vi "WRITE_P.vi"(8 "error in (no error)":errorcluster, 10 "productos 2":T1(array[cluster])) -> (0 "error out":errorcluster)   [LabVIEW 2020, in "Productos.lvlib"]
uses:
  Productos.lvlib
  <vilib>/Utility/xml.llb/Write to XML File(string).vi
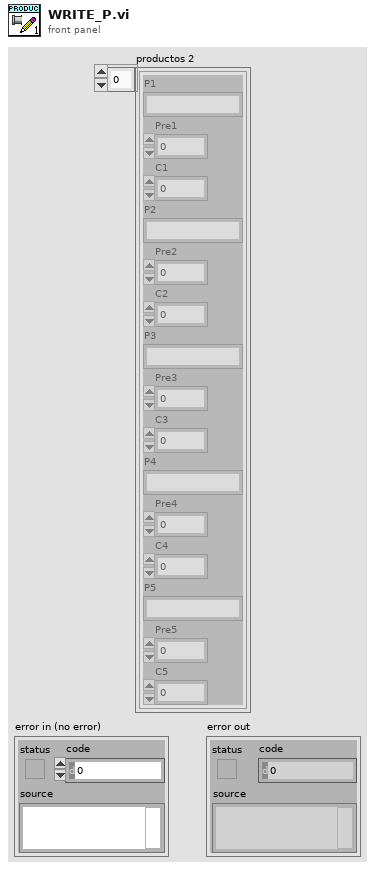
[diagram p1: front panel]
types:
  T1 = cluster{"P1":string, "Pre1":dbl, "C1":dbl, "P2":string, "Pre2":dbl, "C2":dbl, "P3":string, "Pre3":dbl, "C3":dbl, "P4":string, "Pre4":dbl, "C4":dbl, "P5":string, "Pre5":dbl, "C5":dbl}[]
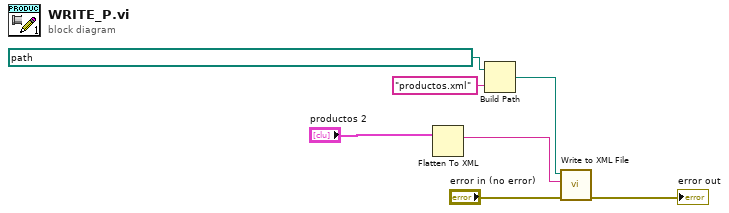
[diagram p0: block diagram]
diagram:
  n1 = Flatten To XML(6:"productos 2") -> (2:w5:string)
  n2 = Build Path(base path=path "C:/Users/Ymata/Desktop/séptimo/labview 7mo/Proyecto máuina/Proyecto-maquina", name or relative path="productos.xml") -> (appended path=w2:path)
  n3 = call-poly <vilib>:"Write to XML File.vi"("error in (no error)"="error in (no error)", "XML Input"=w5, "XML File Path"=w2) -> ("error out"=→"error out":errorcluster)  [unwired: 6 in, 2 out]
